vi "Medidorphase.vi"() -> (0 "V phase 3":dynamicdata(graph), 1 "V phase 2":dynamicdata(graph), 2 "V phase 1":dynamicdata(graph), 3 "I phase 2":dynamicdata(graph), 4 "I phase 3":dynamicdata(graph), 5 "I phase 1":dynamicdata(graph), 6 "time":dynamicdata(graph))   [LabVIEW 2025]
panel:
  out "Fase c":string[][](table)
  out "Fase b":string[][](table)
  out "Fase a":string[][](table)
  out "time":string[][](table)
  out "Waveform Graph":dynamicdata(graph)
  out "all data":string[][](table)
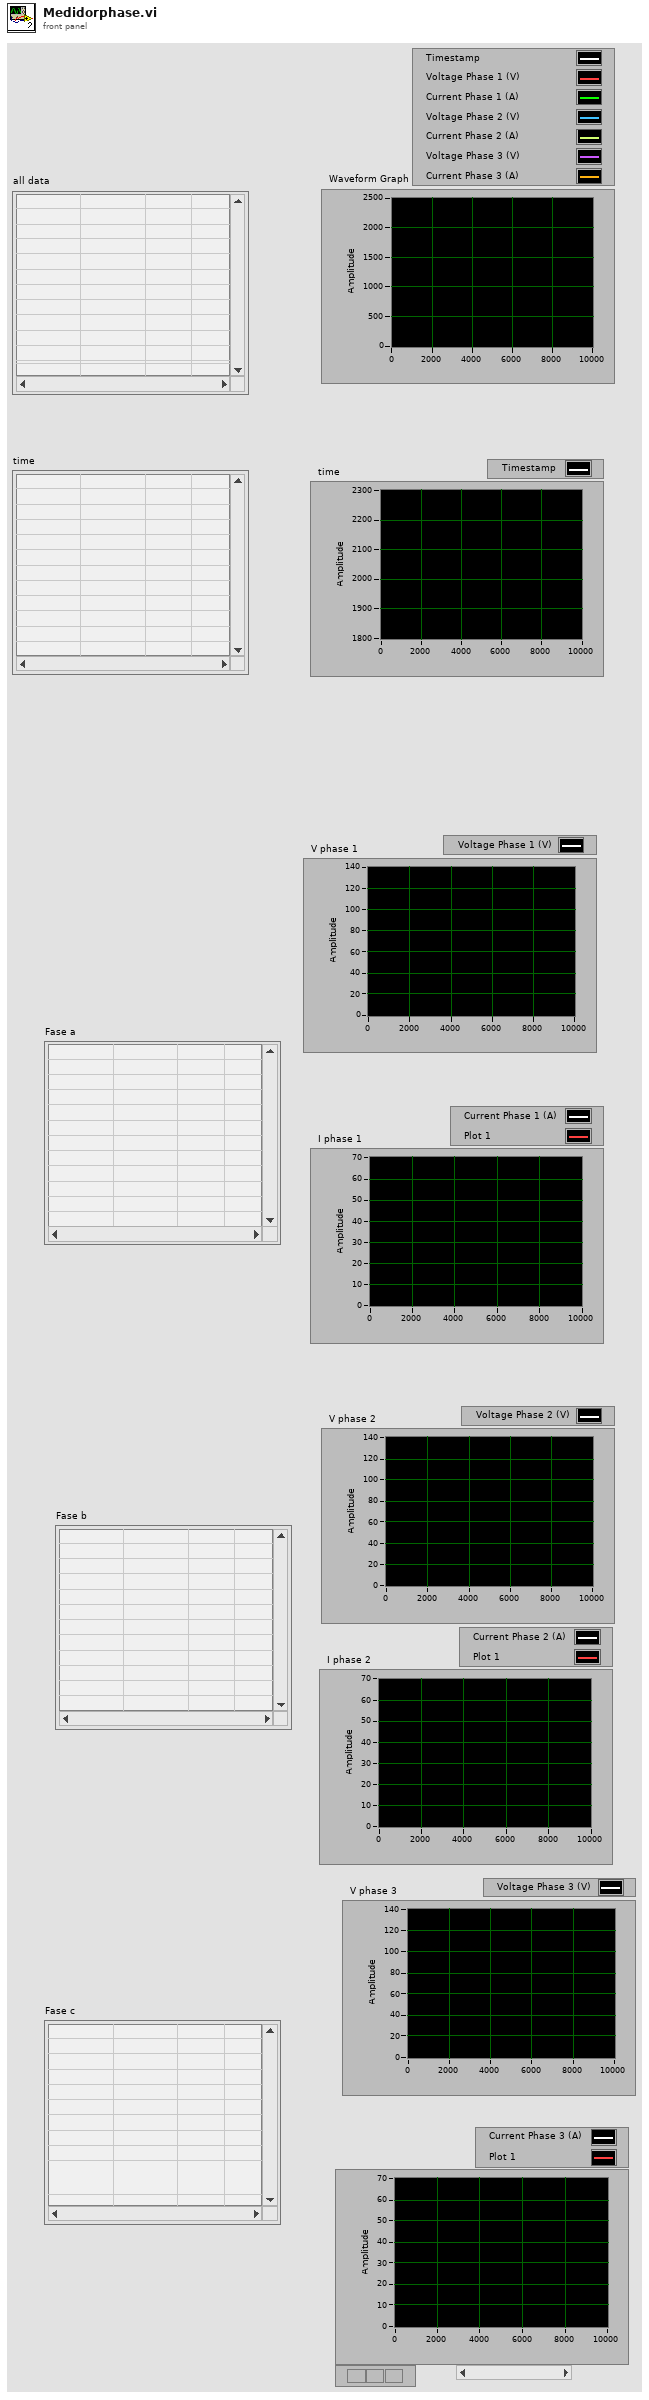
[diagram p1: front panel]
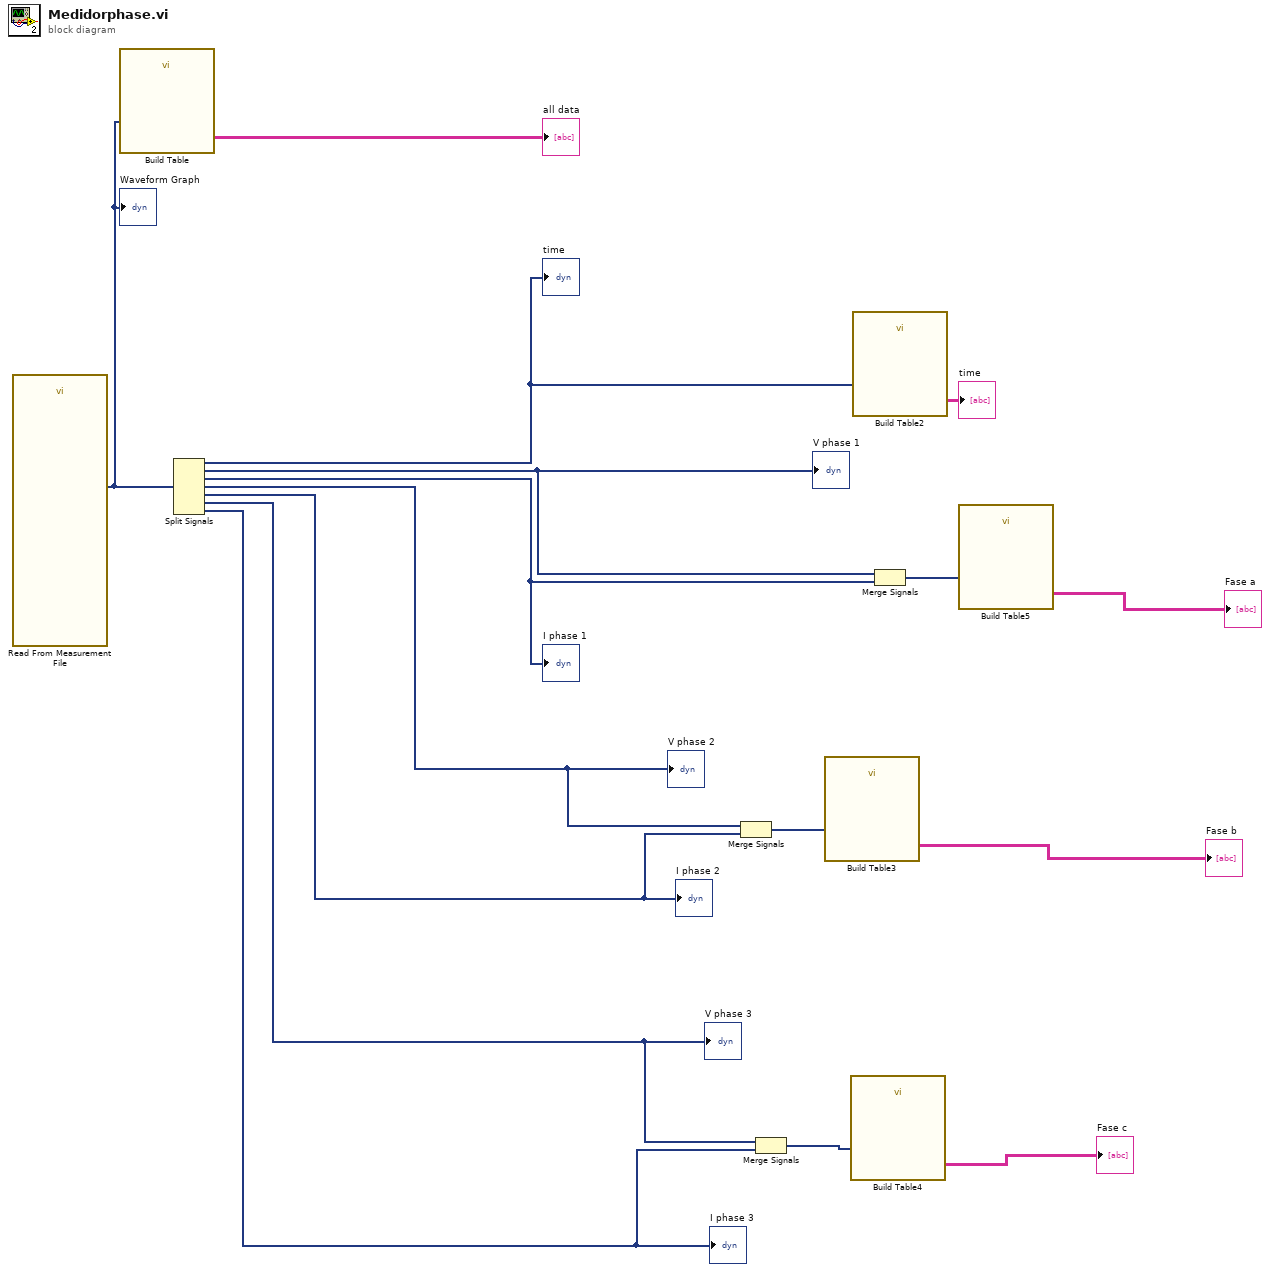
[diagram p0: block diagram]
diagram:
  n1 = call "Read From Measurement File"() -> ("Signals"=w15:dynamicdata)  [unwired: 6 in, 5 out]
  "Waveform Graph" <- w15
  n2 = call "Build Table"("Signals"=w15) -> ("Table"=→"all data":string[][])  [unwired: 4 in, 6 out]
  n3 = Split Signals(w15) -> (w13:dynamicdata, w9:dynamicdata, w10:dynamicdata, w6:dynamicdata, w5:dynamicdata, w2:dynamicdata, w1:dynamicdata)  [unwired: 7 in]
  "time" <- w13
  "V phase 1" <- w9
  "I phase 1" <- w10
  "V phase 2" <- w6
  "I phase 2" <- w5
  "V phase 3" <- w2
  "I phase 3" <- w1
  n4 = Merge Signals(w6, w5) -> (w8:dynamicdata)
  n5 = Merge Signals(w2, w1) -> (w4:dynamicdata)
  n6 = call "Build Table3"("Signals"=w8) -> ("Table"=→"Fase b":string[][])  [unwired: 4 in, 6 out]
  n7 = call "Build Table4"("Signals"=w4) -> ("Table"=→"Fase c":string[][])  [unwired: 4 in, 6 out]
  n8 = call "Build Table2"("Signals"=w13) -> ("Table"=→"time":string[][])  [unwired: 4 in, 6 out]
  n9 = Merge Signals(w9, w10) -> (w12:dynamicdata)
  n10 = call "Build Table5"("Signals"=w12) -> ("Table"=→"Fase a":string[][])  [unwired: 4 in, 6 out]
